vi "cm2nm_read_session_data_file.vi"(2 "TopLevelDataFilePath":path, 3 "Session_data_base":path) -> (1 "Session Information":T1)   [LabVIEW 2011]
doc: "Read the session in and parse it into session information. Write the file if there are changes. Currently disables read from meta data files. operator needs to be in charge of this action."
uses:
  cm2nm_sample_set.ctl
  cm2nm_coordinate_information_v2.ctl
  Instrument_type_enum_v2.ctl
  <vilib>/Utility/xml.llb/Read From XML File(string).vi
panel:
  out "Array name":string[](array[string])
  out "String":string
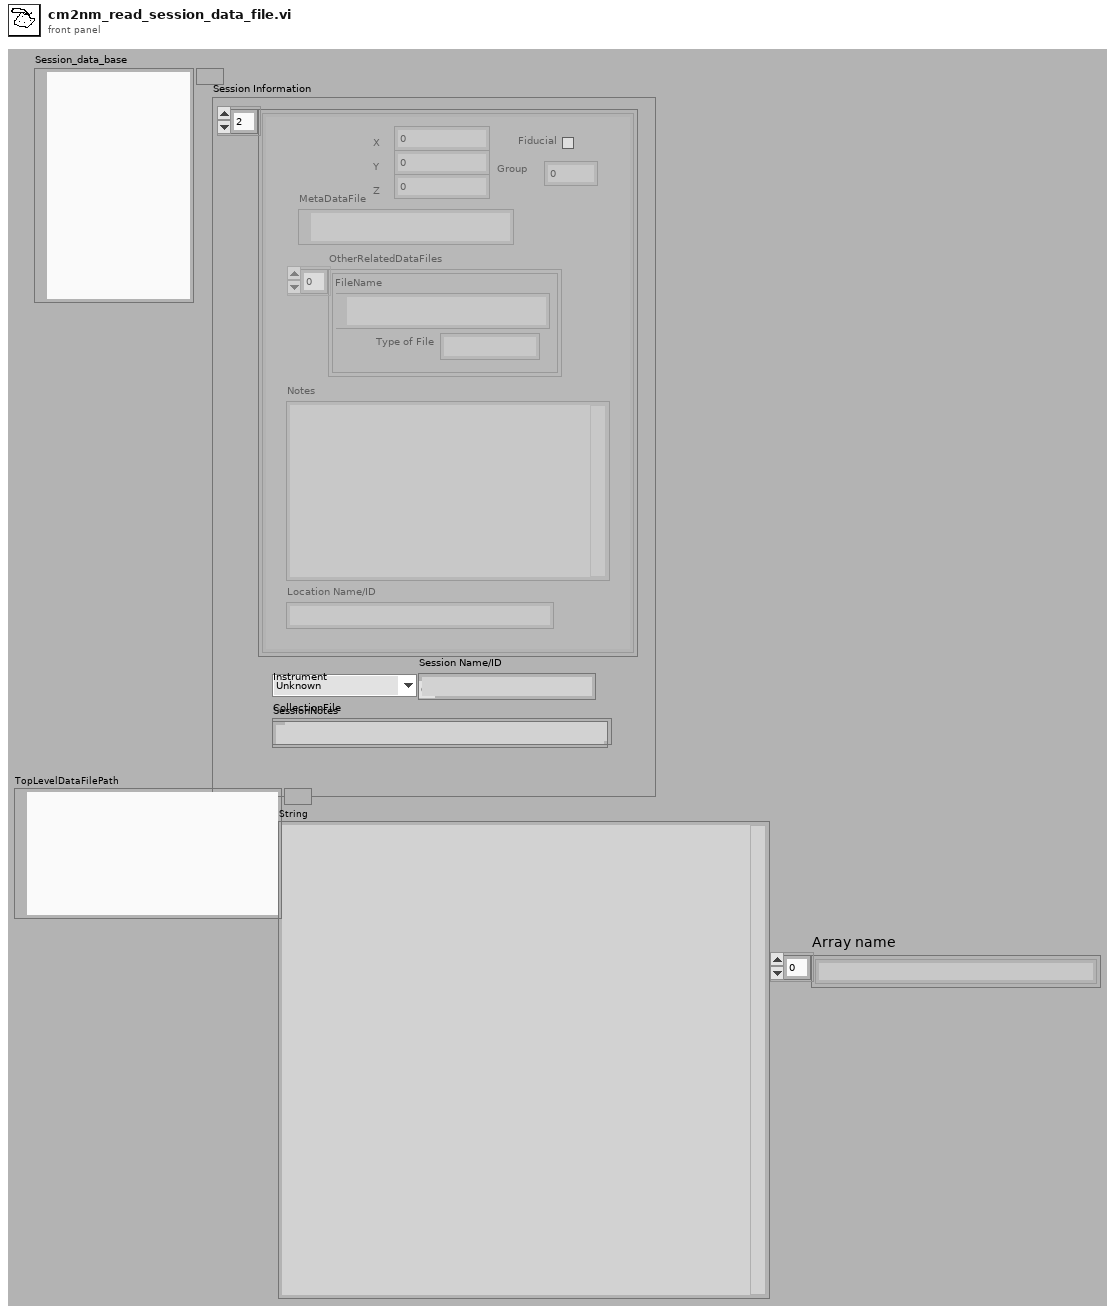
[diagram p1: front panel]
types:
  T1 = typedef "cm2nm_sample_set.ctl" = cluster{"CollectionOfPoints":T2[], "Instrument":T3, "CollectionFile":path, "Session Name/ID":string, "SessionNotes":string}
  T2 = typedef "cm2nm_coordinate_information_v2.ctl" = cluster{"MetaDataFile":path, "X":dbl, "Y":dbl, "Z":dbl, "Group":i32, "Rotation":dbl[unit], "Fiducial":bool, "Magnification":dbl, "Working_Distance":dbl, "Notes":string, "Location Name/ID":string, "OtherRelatedDataFiles":cluster{"Type of File":string, "FileName":path}[], "Available":bool}
  T3 = typedef "Instrument_type_enum_v2.ctl" = enum16{"Unknown", "Philips FEI SEM IRC", "JEOL 7000F EML_MFC", "MXRD MFC", "JEOL_EPMA"}
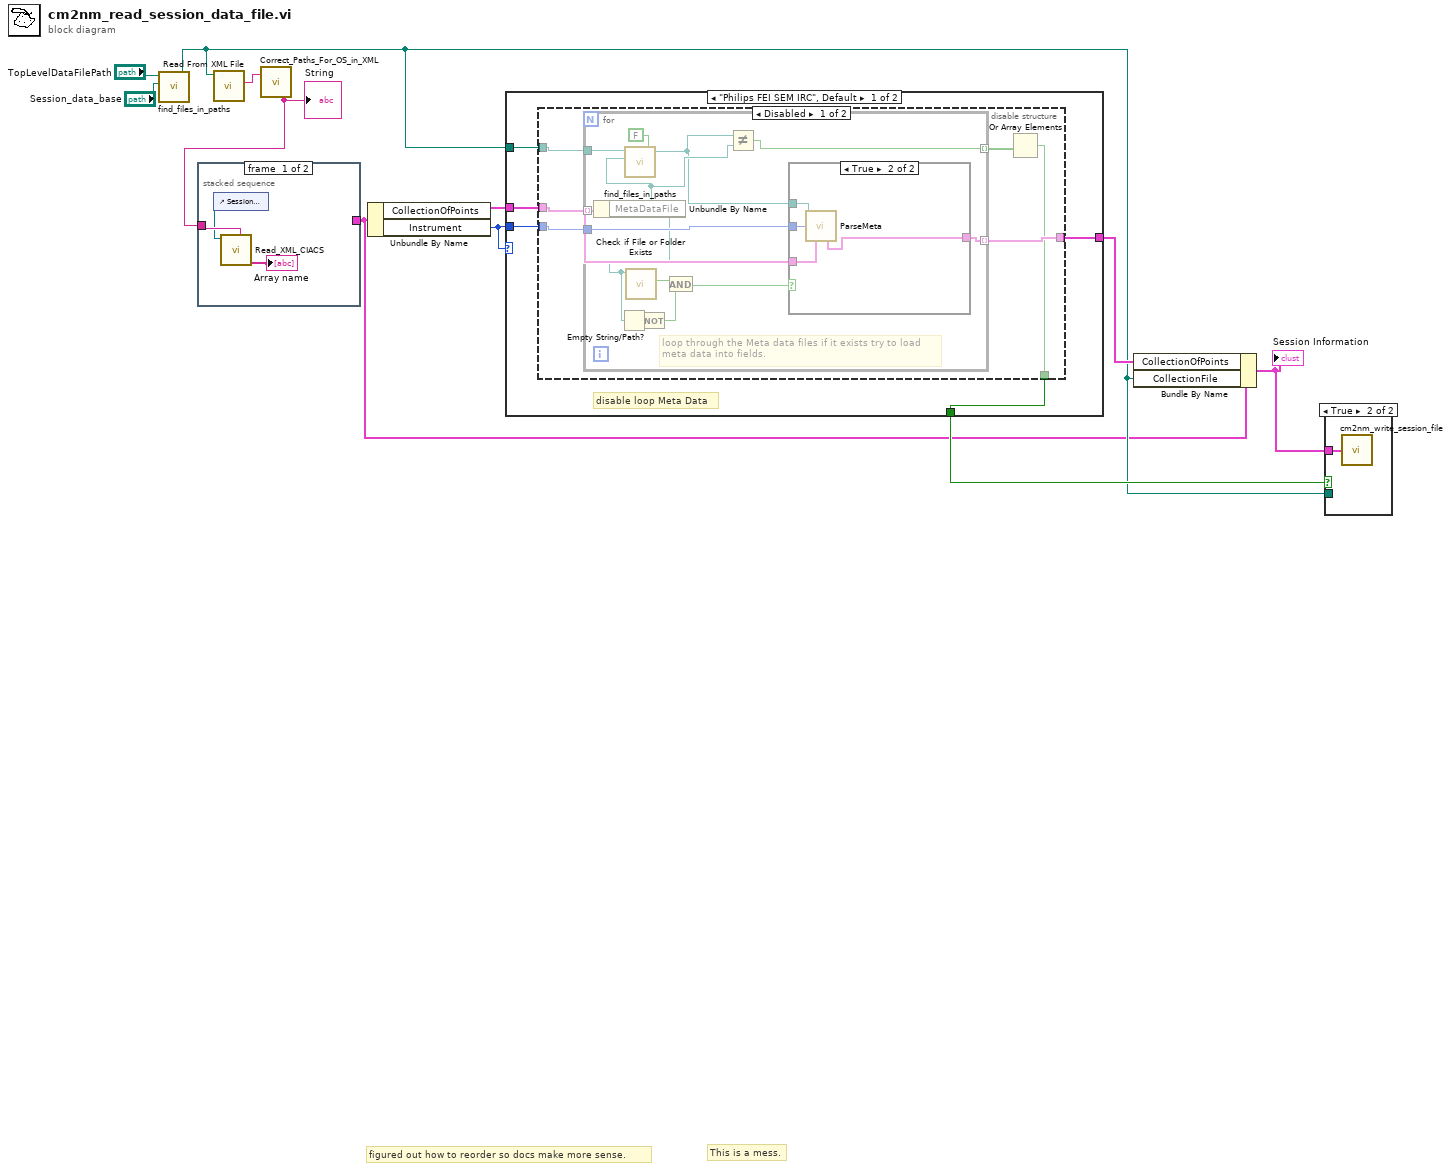
[diagram p0: block diagram]
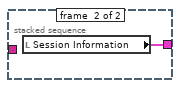
[diagram p2: hidden frame]
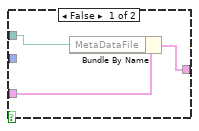
[diagram p4: hidden frame]
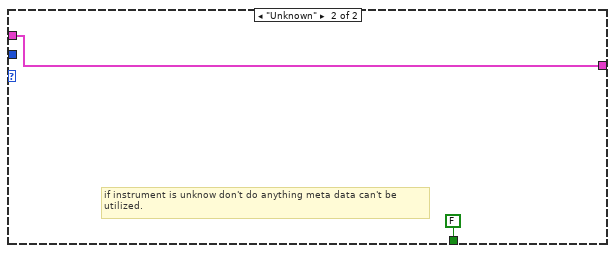
[diagram p6: hidden frame]
diagram:
  # "This is a mess."
  # "figured out how to reorder so docs make more sense."
  n1 = call "find_files_in_paths.vi"("TopLevelDataFilePath"="TopLevelDataFilePath", "File2Find"="Session_data_base") -> ("Path"=w4:path)  [unwired: 4 in, 1 out]
  n2 = call-poly <vilib>:"Read From XML File.vi"("XML File Path"=w4) -> ("XML Elements"=w7:string)  [unwired: 1 in, 9 out]
  n3 = call "Correct_Paths_For_OS_in_XML.vi"("XML Elements"=w7) -> ("String"=w3:string)  [unwired: 1 in]
  "String" <- w3
  n4 = stacked-sequence {
    tunnel: w3 -> [w14 _]
    tunnel: [_ w15] -> w2
    frame #0 {
      n5 = control-ref of="Session Information"() -> (w13:refnum<vi>)
      n6 = call "Read_XML_CIACS.vi"("ReferenceToControl"=w13, "XML_Cluster_String"=w14) -> ("Array"=→"Array name":string[])  [unwired: 4 in, 3 out]
    }
    frame #1 {
      n7 = local read "Session Information"() -> (w15:T1)
    }
  }
  n8 = Unbundle By Name(w2) -> ("CollectionOfPoints"=w11:T2[], "Instrument"=w9:T3)
  n9 = case shown="\"Philips FEI SEM IRC\", Default" w9 {
    tunnel: w11 -> [w20 w48]
    tunnel: w9 -> [w19 _]
    tunnel: [w18 w48] -> w10
    tunnel: w4 -> [w17 _]
    tunnel: [w16 FALSE] -> w8
    frame "Philips FEI SEM IRC", Default {
      # "disable loop Meta Data"
      n10 = disable-structure shown="Disabled" {
        disable-tunnel: w20 -> [w26 w46]
        disable-tunnel: w19 -> [w25 _]
        disable-tunnel: [w24 w46] -> w18
        disable-tunnel: w17 -> [w22 _]
        disable-tunnel: [w21 _] -> w16
        frame Disabled {
          n11 = for {
            tunnel: w26 -> [w37] mode=indexing
            tunnel: w25 -> [w38]
            tunnel: [w36] -> w24 mode=indexing
            tunnel: w22 -> [w31]
            tunnel: [w27] -> w23 mode=indexing
            # "loop through the Meta data files if it exists try to load\nmeta data into fields."
            n12 = Unbundle By Name(w37) -> ("MetaDataFile"=w29:path)
            n13 = Empty String/Path?(string/path=w29) -> (empty?=w35:bool)
            n14 = call "find_files_in_paths.vi"("TopLevelDataFilePath"=w31, "File2Find"=w29, "PromptFormissingFile"=FALSE) -> ("Path"=w28:path)  [unwired: 3 in, 1 out]
            n15 = call <vilib>:"Check if File or Folder Exists.vi"("path"=w29) -> ("file or folder exists?"=w32:bool)  [unwired: 1 in, 9 out]
            n16 = Not(x=w35) -> (.not. x?=w33:bool)
            n17 = And(x=w32, y=w33) -> (x .and. y?=w34:bool)
            n18 = Not Equal?(x=w28, y=w29) -> (x != y?=w27:bool)
            n19 = case shown="True" w34 {
              tunnel: w38 -> [_ w45]
              tunnel: w28 -> [w40 w44]
              tunnel: w37 -> [w41 w43]
              tunnel: [w39 w42] -> w36
              frame False {
                n20 = Bundle By Name(cluster=w41, "MetaDataFile"=w40) -> (w39:T2)
              }
              frame True {
                n21 = call "ParseMeta.vi"("Path"=w44, "Instrument"=w45, "Spot_info_in"=w43) -> ("Spot_info_out"=w42:T2)  [unwired: 12 out]
              }
            }
          }
          n22 = Or Array Elements(Boolean array=w23) -> (logical OR=w21:bool)
        }
        frame Enabled {
        }
      }
    }
    frame "Unknown" {
      # "if instrument is unknow don't do anything meta data can't be\nutilized."
    }
  }
  n23 = Bundle By Name(cluster=w2, "CollectionOfPoints"=w10, "CollectionFile"=w4) -> (w1:T1)
  "Session Information" <- w1
  n24 = case shown="True" w8 {
    tunnel: w4 -> [_ _]
    tunnel: w1 -> [_ w49]
    frame False {
    }
    frame True {
      n25 = call "cm2nm_write_session_file.vi"("Session Information"=w49) -> ()  [unwired: 1 out]
    }
  }
